vi "destroy.vi"(8 "error in (no error)":errorcluster, 11 "librarian_sm in":refnum<class "client.lvclass">) -> (0 "error out":errorcluster, 3 "librarian_sm out":refnum<class "client.lvclass">)   [LabVIEW 2020, in "client.lvclass"]
uses:
  client.lvclass
  client.lvclass/client.ctl
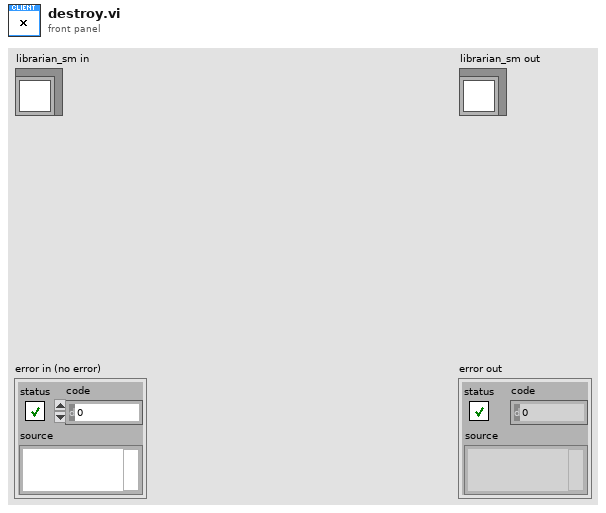
[diagram p1: front panel]
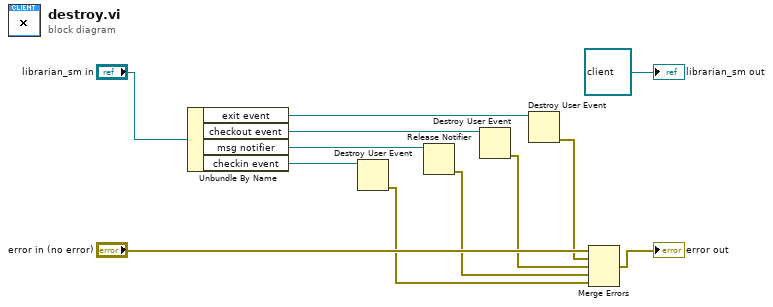
[diagram p0: block diagram]
diagram:
  n1 = Unbundle By Name("librarian_sm in") -> ("exit event"=w11:refnum<user-event>, "checkout event"=w6:refnum<user-event>, "msg notifier"=w4:refnum<notifier>, "checkin event"=w3:refnum<user-event>)
  n2 = Destroy User Event(user event=w3) -> (error out=w1:errorcluster)  [unwired: 1 in]
  n3 = Release Notifier(notifier=w4) -> (error out=w2:errorcluster)  [unwired: 2 in, 2 out]
  n4 = Destroy User Event(user event=w6) -> (error out=w5:errorcluster)  [unwired: 1 in]
  n5 = Destroy User Event(user event=w11) -> (error out=w8:errorcluster)  [unwired: 1 in]
  n6 = Merge Errors("error in (no error)", w8, w5, w2, w1) -> (→"error out":errorcluster)
  "librarian_sm out" <- refnum<class "client.lvclass"> refnum ("librarian_sm out")
